vi "Get.vi"(8 "error in":errorcluster) -> (0 "error out":errorcluster, 3 "Master Reference":T1)   [LabVIEW 2026, in "UserEventRecorder.lvlib" / "VI Reference Management.lvlib"]
doc: "Get the master reference for the cloneable Main VI.\n_____\nBased on DQMH Dev Tools: Project Template 7.1.2.1547."
uses:
  VI Reference Management.lvlib
  Main VI Type--strict_vi_ref.ctl
  <vilib>/Delacor/Delacor QMH/Libraries/Cloneable Module Admin_class/Delacor_lib_QMH_Cloneable Module Admin.lvclass
  Action--enum.ctl
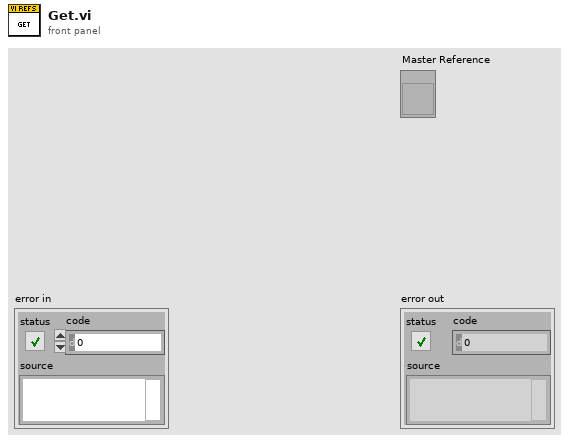
[diagram p1: front panel]
types:
  T1 = typedef "UserEventRecorder.lvlib/VI Reference Management.lvlib/Main VI Type--strict_vi_ref.ctl" = refnum<vi>
  T2 = typedef "UserEventRecorder.lvlib/VI Reference Management.lvlib/Action--enum.ctl" = enum16{"Get", "Create", "Close"}
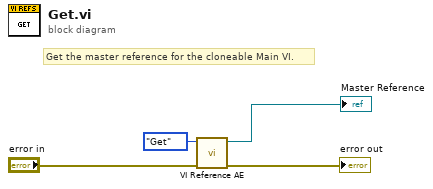
[diagram p0: block diagram]
diagram:
  # "Get the master reference for the cloneable Main VI."
  n1 = call "VI Reference AE.vi"("error in"="error in", "Action"=Action--enum."Get") -> ("error out"=→"error out":errorcluster, "Master Reference"=→"Master Reference":T1)  [unwired: 7 in]
